vi "Root 3 Multiply.vi"(11 "RMS Line to Neutral":dbl) -> (3 "RMS Line to Line":dbl)   [LabVIEW 2018, in "AE75TX Actor.lvlib" / "AE75TX.lvclass"]
uses:
  AE75TX.lvclass
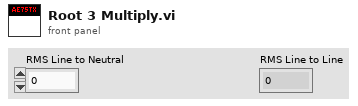
[diagram p1: front panel]
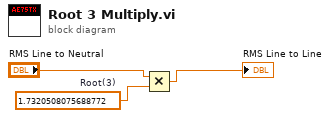
[diagram p0: block diagram]
diagram:
  w1 = 1.7320508075688772  # Root(3)
  n1 = Multiply(x="RMS Line to Neutral", y=w1) -> (x*y=→"RMS Line to Line":dbl)
